vi "AVS_SetPwmOut.vi"(0 "a_hDevice":i32, 7 "a_PortId":u8, 9 "a_Freq":u32, 11 "a_Duty":u8) -> (4 "Output Value":i32)   [LabVIEW 2009]
uses:
  avaspecx64.dll
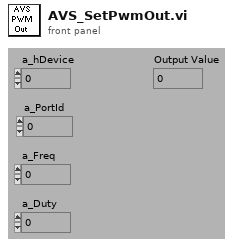
[diagram p1: front panel]
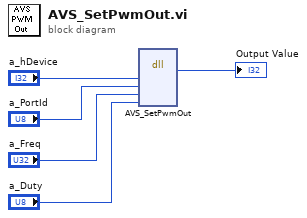
[diagram p0: block diagram]
diagram:
  n1 = dll-call lib="E:/Documents and Settings/mattc/Libraries/Avaspec_Library/trunk/demo_64bit/LabView/LabViewSingleChan/avaspecx64.dll" fn="AVS_SetPwmOut"("a_hDevice"="a_hDevice", "a_PortId"="a_PortId", "a_Freq"="a_Freq", "a_Duty"="a_Duty") -> ("return type"=→"Output Value":i32)  [unwired: 7 in, 2 out]
